vi "name_dipole_voltage.vi"(0 "Num files":i32=1, 2 "iteration number":i32, 3 "Dipole average settings":T1) -> (1 "Voltage name":dbl)   [LabVIEW 2016]
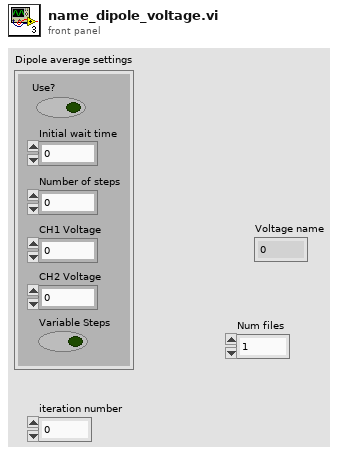
[diagram p1: front panel]
types:
  T1 = cluster{"Initial wait time":dbl, "Number of steps":i32, "CH1 Voltage":dbl, "Use?":bool, "CH2 Voltage":dbl, "Variable Steps":bool}
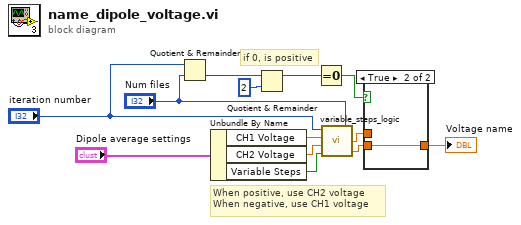
[diagram p0: block diagram]
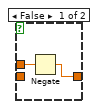
[diagram p2: hidden frame]
diagram:
  # "if 0, is positive"
  # "When positive, use CH2 voltage\nWhen negative, use CH1 voltage"
  n1 = Quotient & Remainder(x="iteration number", y="Num files") -> (floor(x/y)=w13:i32)  [unwired: 1 out]
  n2 = Unbundle By Name("Dipole average settings") -> ("CH1 Voltage"=w12:dbl, "CH2 Voltage"=w11:dbl, "Variable Steps"=w10:bool)
  n3 = Quotient & Remainder(x=w13, y=2) -> (x-y*floor(x/y)=w9:i32)  [unwired: 1 out]
  n4 = Equal To 0?(x=w9) -> (x = 0?=w5:bool)
  n5 = call "variable_steps_logic.vi"("Num files"="Num files", "Variable Steps"=w10, "Voltage 2"=w11, "Voltage 1"=w12, "iteration number"="iteration number") -> ("Returned Voltage 2"=w6:dbl, "Returned Voltage 1"=w7:dbl)
  n6 = case shown="True" w5 {
    tunnel: [w14 w16] -> w4
    tunnel: w6 -> [_ w16]
    tunnel: w7 -> [w15 _]
    frame False {
      n7 = Negate(x=w15) -> (-x=w14:dbl)
    }
    frame True {
    }
  }
  "Voltage name" <- w4
